vi "test.vi"() -> ()   [LabVIEW 2014]
uses:
  <vilib>/Instr/_visa.llb/VISA Configure Serial Port (Instr).vi
panel:
  in  "VISA resource name":refnum<visa-resource-name>
  out "Threshold sent":bool
  out "Pass Ack":bool
  out "password is wrong":bool
  in  "Tab Control":enum32{"Page 1", "Page 2", "Page 3"}(tab)
  in  "Password":string
  in  "Threshold":string
  out "Iteration":i32
  in  "Reset":bool
  out "Reset#":i32
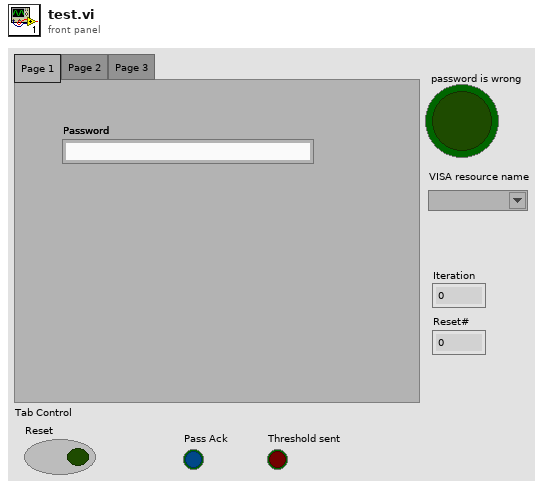
[diagram p1: front panel]
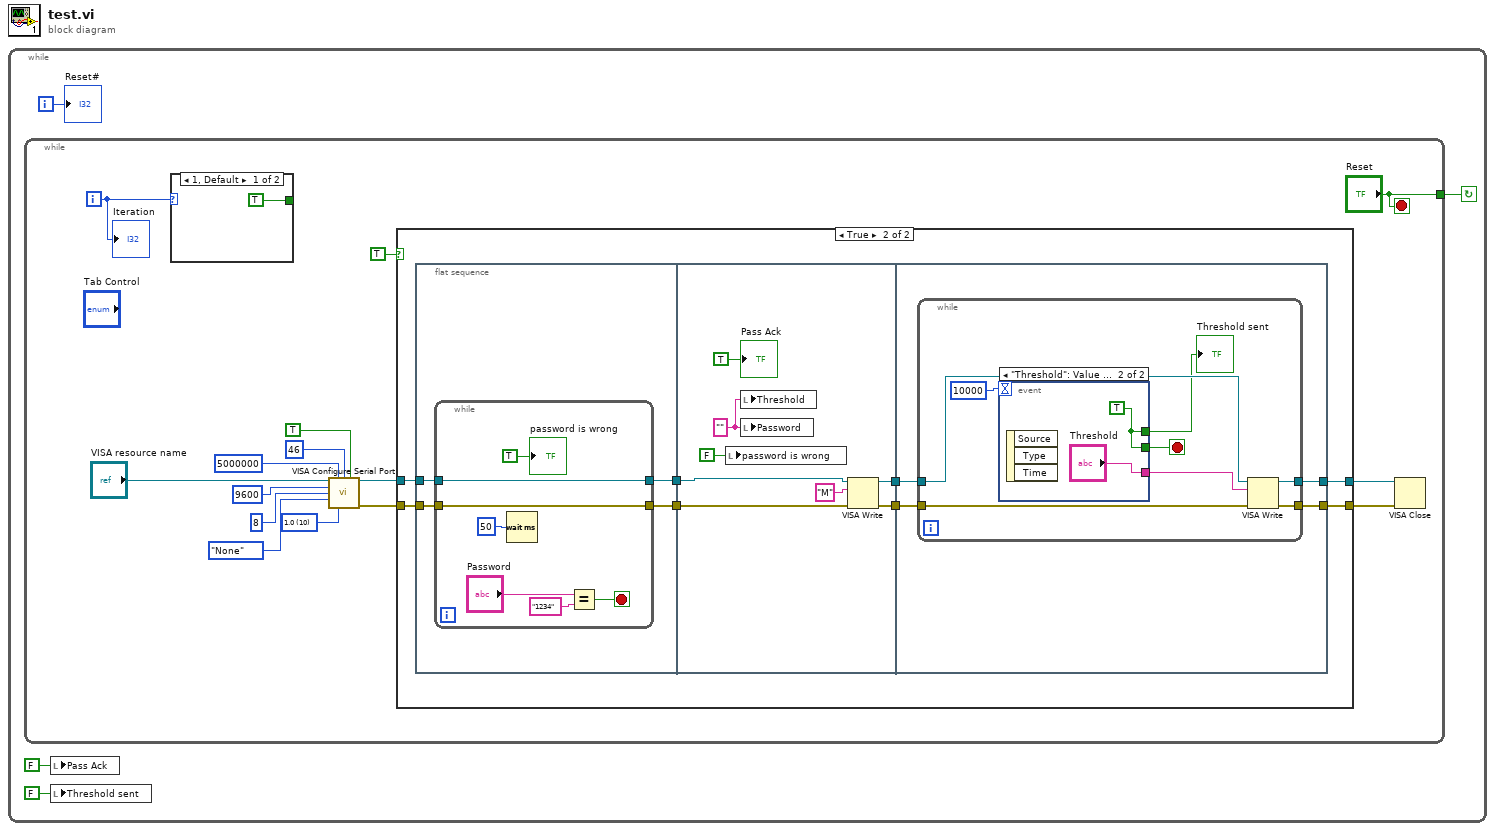
[diagram p0: block diagram]
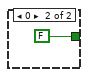
[diagram p2: hidden frame]
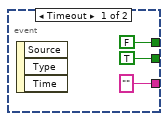
[diagram p4: hidden frame]
diagram:
  n1 = while {
    i -> [w4]
    stop <- w3 continue-if-true
    n2 = while {
      tunnel: ["Reset"] -> w3
      i -> [w9]
      stop <- "Reset" stop-if-true
      w16 = u16 10 items=["1.0"=10, "1.5"=15, "2.0"=20] ("stop bits (10: 1 bit)")
      n3 = case shown="1, Default" w9 {
        tunnel: [TRUE FALSE] -> _
        frame 1, Default {
        }
        frame 0 {
        }
      }
      n4 = call-poly "VISA Configure Serial Port"("VISA resource name"="VISA resource name", "timeout (10sec)"=u32 5000000, "termination char\n(0xA = '\\n' = LF)"=u8 46 ("termination char\n(0xA = '\\n' = LF)"), "Enable Termination\nChar (T)"=TRUE ("Enable Termination\nChar (T)"), "baud rate (9600)"=u32 9600, "data bits (8)"=u16 8, "parity (0:none)"=enum16{"None", "Odd", "Even", "Mark", "Space"}."None", "stop bits (10: 1 bit)"=w16) -> ("VISA resource name out"=w11:refnum<visa-resource-name>, "error out"=w10:errorcluster)  [unwired: 6 in]
      n5 = case shown="True" TRUE {
        tunnel: w10 -> [w23 w31]
        tunnel: [w22 w29] -> w5
        tunnel: [w23 w28] -> w6
        tunnel: w11 -> [w22 w30]
        frame False {
        }
        frame True {
          n6 = flat-sequence {
            tunnel: w31 -> [w35]
            tunnel: w30 -> [w34]
            tunnel: [w33] -> w27
            tunnel: [w32] -> w26
            tunnel: w27 -> [w50]
            tunnel: w26 -> [w49]
            tunnel: [w48] -> w25
            tunnel: [w47] -> w24
            tunnel: [w53] -> w29
            tunnel: [w52] -> w28
            tunnel: w25 -> [w54]
            tunnel: w24 -> [w51]
            frame #0 {
              n7 = while {
                tunnel: w35 -> [w40]
                tunnel: w34 -> [w39]
                tunnel: [w40] -> w33
                tunnel: [w39] -> w32
                stop <- w41 stop-if-true
                n8 = Wait (ms)(milliseconds to wait=u32 50) -> ()  [unwired: 1 out]
                n9 = Equal?(x="Password", y="1234") -> (x = y?=w41:bool)
                "password is wrong" <- TRUE
              }
            }
            frame #1 {
              w43 = "" ("Password")
              n10 = local write "password is wrong"(FALSE) -> ()
              n11 = local write "Threshold"(w43) -> ()
              n12 = local write "Password"(w43) -> ()
              n13 = VISA Write(VISA resource name=w49, write buffer="M", error in (no error)=w50) -> (VISA resource name out=w48:refnum<visa-resource-name>, error out=w47:errorcluster)  [unwired: 1 out]
              "Pass Ack" <- TRUE ("Pass Ack")
            }
            frame #2 {
              n14 = while {
                tunnel: w54 -> [w62]
                tunnel: [w61] -> w53
                tunnel: [w60] -> w52
                tunnel: w51 -> [w59]
                stop <- w56 stop-if-true
                n15 = event shown="[1] \"Threshold\": Value Change" {
                  selector: _ -> [_ _]
                  dyn-events: _ -> [_ _]
                  timeout: 10000 -> [_ _]
                  tunnel: [TRUE w66] -> w56
                  tunnel: ["" "Threshold"] -> w58
                  tunnel: [FALSE w66] -> w55
                  event Timeout {
                    n16 = event-data() -> ()  [unwired: 1 in, 3 out]
                  }
                  event "Threshold": Value Change {
                    w66 = TRUE
                    n17 = event-data() -> ()  [unwired: 1 in, 3 out]
                  }
                }
                "Threshold sent" <- w55
                n18 = VISA Write(VISA resource name=w62, write buffer=w58, error in (no error)=w59) -> (VISA resource name out=w61:refnum<visa-resource-name>, error out=w60:errorcluster)  [unwired: 1 out]
              }
            }
          }
        }
      }
      n19 = VISA Close(VISA resource name=w5, error in (no error)=w6) -> ()  [unwired: 1 out]
      "Iteration" <- w9
    }
    n20 = local write "Pass Ack"(FALSE) -> ()
    n21 = local write "Threshold sent"(FALSE ("Pass Ack")) -> ()
    "Reset#" <- w4
  }
